vi "Initialize.vi"(6 "Startup delay (0 ms)":u32, 8 "error in (no error)":errorcluster, 9 "Reset (False)":bool, 10 "ID Query (True)":bool=TRUE, 11 "VISA resource name":refnum<visa-resource-name>) -> (0 "error out":errorcluster, 2 "ID":string, 3 "VISA resource name out":refnum<visa-resource-name>)   [LabVIEW 2020, in "QuPMXdriver.lvlib"]
doc: "Establishes communication with the Multiplexer, performs an identification query and/or an instrument reset. Call this VI before calling other instrument driver VIs for this instrument. Generally, you need to call the <b>Initialize</b> VI only once at the beginning of an application."
uses:
  QuPMXdriver.lvlib
panel:
  # "(c) 2021 Czech Metrology Institute.  ALL RIGHTS RESERVED."
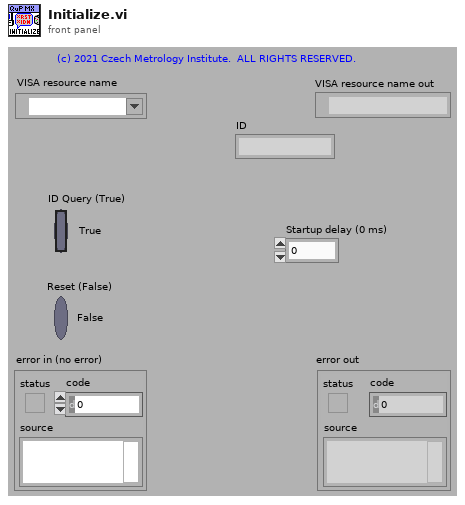
[diagram p1: front panel]
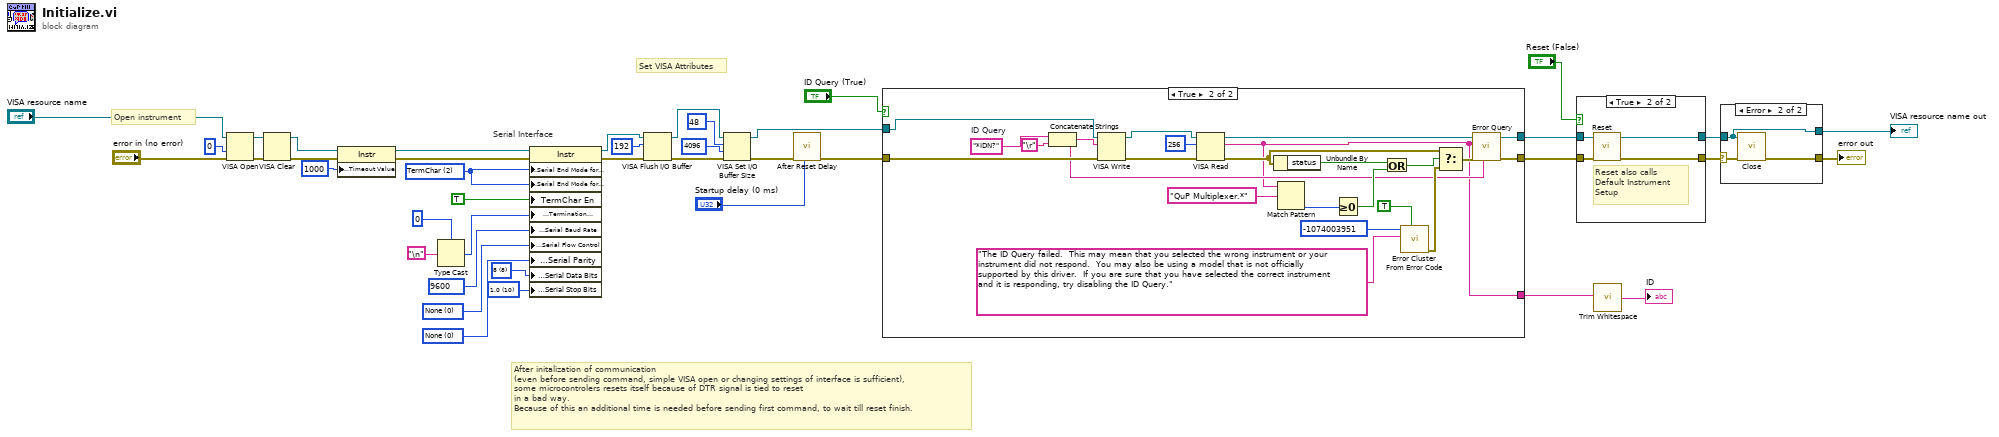
[diagram p0: block diagram]
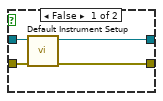
[diagram p3: hidden frame]
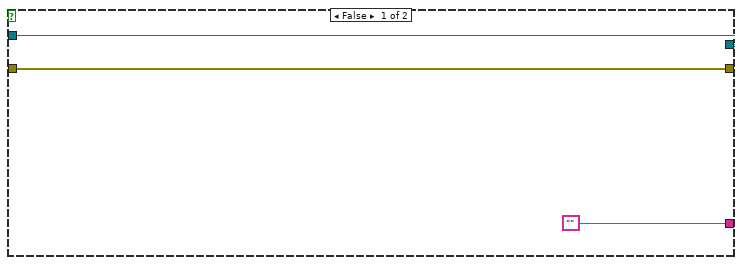
[diagram p4: hidden frame]
diagram:
  w13 = u32 9600 items=["300"=300, "600"=600, "1200"=1200, "2400"=2400, "4800"=4800, "9600"=9600, "19200"=19200] ("Baud Rate")
  w9 = u16 0 items=["None", "Odd", "Even", "Mark", "Space"] ("Parity")
  w12 = u16 8 items=["7"=7, "8"=8] ("Data Bits")
  w11 = u16 10 items=["1.0"=10, "1.5"=15, "2.0"=20] ("Stop Bits")
  w10 = u16 0 items=["None", "XON/XOFF", "RTS/CTS", "XON/XOFF & RTS/CTS", "DTR/DSR", "XON/XOFF & DTR/DSR"] ("Flow Control")
  w15 = u16 2 items=["None", "LastBit", "TermChar"] ("Serial Settings:Serial End Mode for Reads")
  # "After initalization of communication\n(even before sending command, simple VISA open or changing settings of interface is sufficient),\nsome microcontrolers resets itself because of DTR signal is tied to reset\nin a bad way.\nBecause of this an additional time is needed before sending first command, to wait till reset finish."
  # "Serial Interface"
  # "Set VISA Attributes"
  # "Open instrument"
  n1 = VISA Open(access mode=u32 0, error in (no error)="error in (no error)", VISA resource name="VISA resource name") -> (VISA resource name=w32:refnum<visa-resource-name>, error out=w31:errorcluster)  [unwired: 2 in]
  n2 = VISA Clear(VISA resource name=w32, error in (no error)=w31) -> (VISA resource name out=w30:refnum<visa-resource-name>, error out=w29:errorcluster)
  n3 = property class="Instr"(reference=w30, error in=w29, "General Settings:Timeout Value"=u32 1000) -> (reference out=w35:refnum<visa-resource-name>, error out=w34:errorcluster)
  n4 = Type Cast(type=u8 0, x="\n" ("Line Feed Constant")) -> (*(type *) &x=w14:u8)
  n5 = property class="Instr"(reference=w35, error in=w34, "Serial Settings:Serial End Mode for Reads"=w15, "Serial Settings:Serial End Mode for Writes"=w15, "TermChar En"=TRUE ("Message Based Settings:Termination Character Enable"), "Message Based Settings:Termination Character"=w14, "Serial Settings:Serial Baud Rate"=w13, "Serial Settings:Serial Flow Control"=w10, "Serial Settings:Serial Parity"=w9, "Serial Settings:Serial Data Bits"=w12, "Serial Settings:Serial Stop Bits"=w11) -> (reference out=w21:refnum<visa-resource-name>, error out=w23:errorcluster)
  n6 = VISA Flush I/O Buffer(VISA resource name=w21, mask (16)=u16 192, error in (no error)=w23) -> (VISA resource name out=w24:refnum<visa-resource-name>, error out=w22:errorcluster)
  n7 = VISA Set I/O Buffer Size(VISA resource name=w24, mask (16)=u16 48, size (4096)=u32 4096 ("size (0)"), error in (no error)=w22) -> (VISA resource name out=w36:refnum<visa-resource-name>, error out=w7:errorcluster)
  n8 = call "After Reset Delay.vi"("Reset delay (2000 ms)"="Startup delay (0 ms)", "error in"=w7) -> ("error out"=w6:errorcluster)  [unwired: 9 in]
  n9 = case shown="True" "ID Query (True)" {
    tunnel: [w43 w51] -> w1
    tunnel: [w44 w50] -> w2
    tunnel: w36 -> [w44 w66]
    tunnel: w6 -> [w43 w67]
    tunnel: ["" w47] -> w5
    frame False {
    }
    frame True {
      w53 = "*IDN?"  # ID Query
      n10 = Concatenate Strings(w53, "\r") -> (w48:string)
      n11 = VISA Write(VISA resource name=w66, write buffer=w48, error in (no error)=w67) -> (VISA resource name out=w45:refnum<visa-resource-name>, error out=w46:errorcluster)  [unwired: 1 out]
      n12 = VISA Read(VISA resource name=w45, byte count=u32 256, error in (no error)=w46) -> (VISA resource name out=w49:refnum<visa-resource-name>, read buffer=w47:string, error out=w58:errorcluster)  [unwired: 1 out]
      n13 = Unbundle By Name(w58) -> ("status"=w57:bool)
      n14 = Match Pattern(string=w47, regular expression="QuP Multiplexer.*") -> (offset past match=w59:i32)  [unwired: 1 in, 3 out]
      n15 = Greater Or Equal To 0?(x=w59) -> (x >= 0?=w56:bool)
      n16 = Or(x=w57, y=w56) -> (x .or. y?=w55:bool)
      n17 = call <vilib>:"Error Cluster From Error Code.vi"("show call chain? (False)"=TRUE, "error message (\"\")"="The ID Query failed.  This may mean that you selected the wrong instrument or your instrument did not respond.  You may also be using a model that is not officially supported by this driver.  If you are sure that you have selected the correct instrument and it is responding, try disabling the ID Query." ("Source (VI Name)"), "error code (0)"=-1074003951 ("Code")) -> ("error out"=w63:errorcluster)  [unwired: 6 in]
      n18 = Select(t=w58, s=w55, f=w63) -> (s? t:f=w52:errorcluster)
      n19 = call "Error Query.vi"("Last command"=w48, "error in (no error)"=w52, "Read buffer"=w47, "VISA resource name"=w49) -> ("error out"=w51:errorcluster, "VISA resource name out"=w50:refnum<visa-resource-name>)  [unwired: 6 in]
    }
  }
  n20 = case shown="True" "Reset (False)" {
    tunnel: w1 -> [w70 w72]
    tunnel: [w68 w75] -> w25
    tunnel: w2 -> [w71 w73]
    tunnel: [w69 w74] -> w26
    frame False {
      n21 = call "Default Instrument Setup.vi"("error in (no error)"=w70, "VISA resource name"=w71) -> ("error out"=w68:errorcluster, "VISA resource name out"=w69:refnum<visa-resource-name>)  [unwired: 8 in]
    }
    frame True {
      # "Reset also calls Default Instrument Setup"
      n22 = call "Reset.vi"("error in (no error)"=w72, "VISA resource name"=w73) -> ("error out"=w75:errorcluster, "VISA resource name out"=w74:refnum<visa-resource-name>)  [unwired: 8 in]
    }
  }
  n23 = call <vilib>:"Trim Whitespace.vi"("string"=w5) -> ("trimmed string"=→"ID":string)  [unwired: 1 in]
  n24 = case shown="Error" w25 {
    selector: w25 -> [w76 w79]
    tunnel: w26 -> [w77 w78]
    tunnel: [w77 w78] -> w28
    tunnel: [w76 w80] -> w27
    frame No Error {
    }
    frame Error {
      n25 = call "Close.vi"("error in (no error)"=w79, "VISA resource name"=w78) -> ("error out"=w80:errorcluster)  [unwired: 9 in]
    }
  }
  "VISA resource name out" <- w28
  "error out" <- w27
